vi "FABR-Read Header.vi"(0 "Path":path, 11 "error in (no error)":errorcluster) -> (4 "Header":T6, 6 "Params":T1={"Format"=20, "Stimulus"={"Destination"="", "Rep rate (/sec)"=0.0, "Alternate Polarity"=FALSE, "Duration (ms)"=30.0, "Ramp (ms)"=16.0, "Fs (Hz)"=0.0, "Frame size (s)"=30.0}, "Sequence"={"Freq"={"Expression"="", "Step"=80}, "Level"={"Start (dB)"=20, "Stop (dB)"=80, "Step (dB)"=5}, "Order"=enum."Interleaved"}, "Response"={"Gain"=1.0, "Averages"=10000, "Window (ms)"=512.0, "Fs (Hz)"=8.5, "Save raw"=FALSE}, "Reject"=0.0} {"Sequence"."Level"."Start (dB)" step=5; "Response"."Window (ms)" format="%.2f"}, 15 "error out":errorcluster)   [LabVIEW 2020]
uses:
  Typedefs/FABR-Header.ctl
  Threshold Estimation VIs/ABR3-Threshold Estimation Result.ctl
  Typedefs/FABR-Parameters.ctl
  Typedefs/FABR-Stimulus.ctl
  Typedefs/FABR-Sequence.ctl
  Typedefs/FABR-Order.ctl
  Typedefs/FABR-Response.ctl
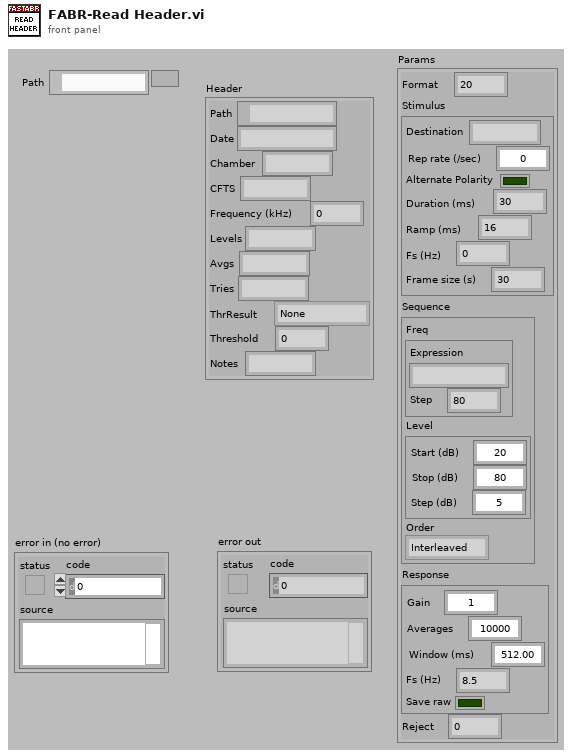
[diagram p1: front panel]
types:
  T1 = typedef "FABR-Parameters.ctl" = cluster{"Format":i32, "Stimulus":T2, "Sequence":T3, "Response":T5, "Reject":dbl}
  T2 = typedef "FABR-Stimulus.ctl" = cluster{"Destination":string, "Rep rate (/sec)":dbl, "Alternate Polarity":bool, "Duration (ms)":dbl, "Ramp (ms)":dbl, "Fs (Hz)":dbl, "Frame size (s)":dbl}
  T3 = typedef "FABR-Sequence.ctl" = cluster{"Freq":cluster{"Expression":string, "Step":i32}, "Level":cluster{"Start (dB)":i32, "Stop (dB)":i32, "Step (dB)":i32}, "Order":T4}
  T4 = typedef "FABR-Order.ctl" = enum16{"Interleaved"}
  T5 = typedef "FABR-Response.ctl" = cluster{"Gain":dbl, "Averages":i32, "Window (ms)":sgl, "Fs (Hz)":dbl, "Save raw":bool}
  T6 = typedef "FABR-Header.ctl" = cluster{"Path":path, "Date":string, "Chamber":string, "CFTS":string, "Frequency (kHz)":dbl, "Levels":string, "Avgs":string, "Tries":string, "ThrResult":T7, "Threshold":dbl, "Notes":string}
  T7 = typedef "ABR3-Threshold Estimation Result.ctl" = enum16{"None", "Power", "Sigmoid", "Power (noisy)", "Suprathreshold", "Invalid"}
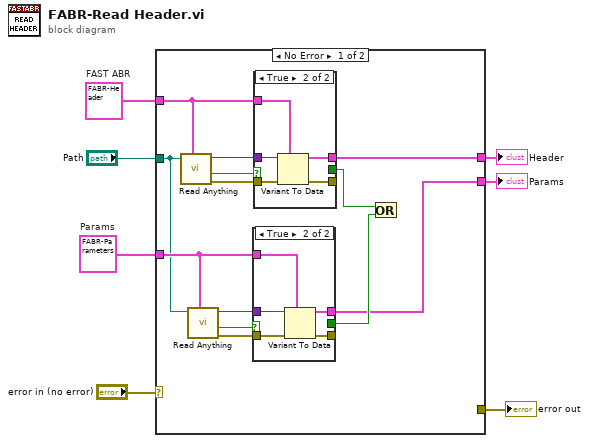
[diagram p0: block diagram]
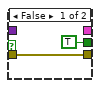
[diagram p2: hidden frame]
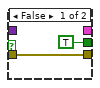
[diagram p3: hidden frame]
diagram:
  w2 = T6 {"Path"=path "", "Date"="", "Chamber"="", "CFTS"="", "Frequency (kHz)"=0.0, "Levels"="", "Avgs"="", "Tries"="", "ThrResult"=enum."None", "Threshold"=0.0, "Notes"=""}  # FAST ABR
  w4 = T1 {"Format"=20, "Stimulus"={"Destination"="", "Rep rate (/sec)"=0.0, "Alternate Polarity"=FALSE, "Duration (ms)"=30.0, "Ramp (ms)"=16.0, "Fs (Hz)"=0.0, "Frame size (s)"=30.0}, "Sequence"={"Freq"={"Expression"="", "Step"=80}, "Level"={"Start (dB)"=20, "Stop (dB)"=80, "Step (dB)"=5}, "Order"=enum."Interleaved"}, "Response"={"Gain"=1.0, "Averages"=10000, "Window (ms)"=512.0, "Fs (Hz)"=8.5, "Save raw"=FALSE}, "Reject"=0.0}  # Params
  n1 = case shown="No Error" "error in (no error)" {
    selector: "error in (no error)" -> [_ w35]
    tunnel: [_ w35] -> w6
    tunnel: "Path" -> [w12 _]
    tunnel: [w9 _] -> w1
    tunnel: w2 -> [w17 _]
    tunnel: w4 -> [w13 _]
    tunnel: [w8 _] -> w3
    frame No Error {
      n2 = call "Read Anything.vi"("Type of Anything"=w17, "Path (dialog)"=w12) -> ("Error Out"=w20:errorcluster, "Found?"=w19:bool, "Anything"=w18:variant)  [unwired: 7 in]
      n3 = call "Read Anything.vi"("Type of Anything"=w13, "Path (dialog)"=w12) -> ("Error Out"=w16:errorcluster, "Found?"=w15:bool, "Anything"=w14:variant)  [unwired: 7 in]
      n4 = case shown="True" w15 {
        tunnel: w16 -> [w22 w27]
        tunnel: w14 -> [_ w26]
        tunnel: w13 -> [_ w25]
        tunnel: [w22 w24] -> _
        tunnel: [_ w23] -> w8
        tunnel: [TRUE _] -> w10
        frame False {
        }
        frame True {
          n5 = Variant To Data(error in=w27, type=w25, Variant=w26) -> (data=w23:T1, error out=w24:errorcluster)
        }
      }
      n6 = case shown="True" w19 {
        tunnel: w20 -> [w29 w34]
        tunnel: w18 -> [_ w33]
        tunnel: w17 -> [_ w32]
        tunnel: [w29 w31] -> _
        tunnel: [_ w30] -> w9
        tunnel: [TRUE _] -> w11
        frame False {
        }
        frame True {
          n7 = Variant To Data(error in=w34, type=w32, Variant=w33) -> (data=w30:T6, error out=w31:errorcluster)
        }
      }
      n8 = Or(x=w11, y=w10) -> ()  [unwired: 1 out]
    }
    frame Error {
    }
  }
  "error out" <- w6
  "Header" <- w1
  "Params" <- w3
